vi "CN740_MODBUS_ASCII.vi"() -> ()   [LabVIEW 2023]
uses:
  <vilib>/Instr/_visa.llb/VISA Configure Serial Port (Instr).vi
panel:
  in  "Hysteresis 1":dbl=100.0 min=0.0 max=300.0 step=0.1 format="%.1f"
  out "Mode ON/OFF":bool
  out "Mode PID":bool
  in  "Switch  Mode":bool
  in  "SV 1":dbl=100.0 min=0.0 max=300.0 step=0.1 format="%.1f"
  out "PV 1":dbl format="%.1f"
  in  "DC Pulse (ON/OFF)":bool
  in  "VISA Controller 1":refnum<visa-resource-name>="COM6"
  in  "Hysteresis":dbl=100.0 min=0.0 max=300.0 step=0.1 format="%.1f"
  in  "Switch Mode":bool
  out "Mode ON/OFF":bool
  out "Mode PID":bool
  in  "DC Pulse (ON/OFF)":bool
  in  "VISA Controller 3":refnum<visa-resource-name>="COM6"
  in  "SV 3":dbl=100.0 min=0.0 max=300.0 step=0.1 format="%.1f"
  out "PV 3":dbl format="%.1f"
  out "Mode ON/OFF":bool
  out "Mode PID":bool
  in  "Switch  Mode":bool
  in  "SV 2":dbl=100.0 min=0.0 max=300.0 step=0.1 format="%.1f"
  out "PV 2":dbl format="%.1f"
  in  "DC Pulse (ON/OFF)":bool
  in  "Hysteresis":dbl=100.0 min=0.0 max=300.0 step=0.1 format="%.1f"
  in  "VISA Controller 2":refnum<visa-resource-name>="COM6"
  in  "stop":bool
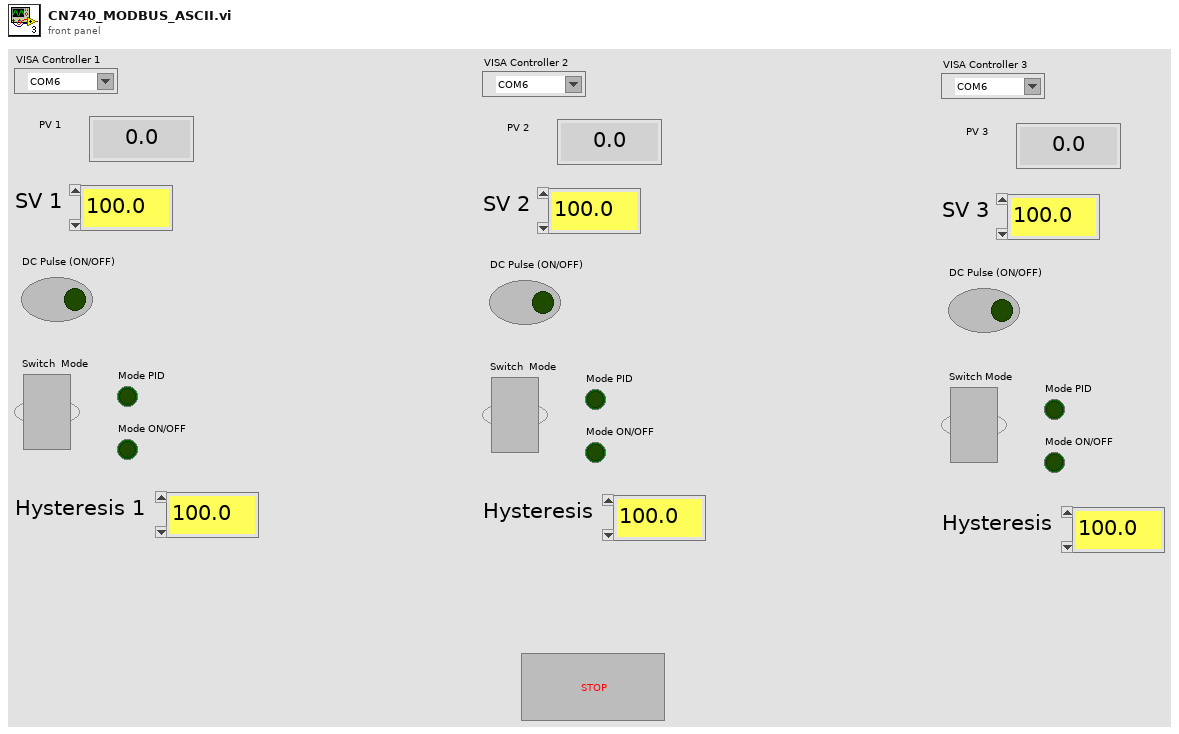
[diagram p1: front panel]
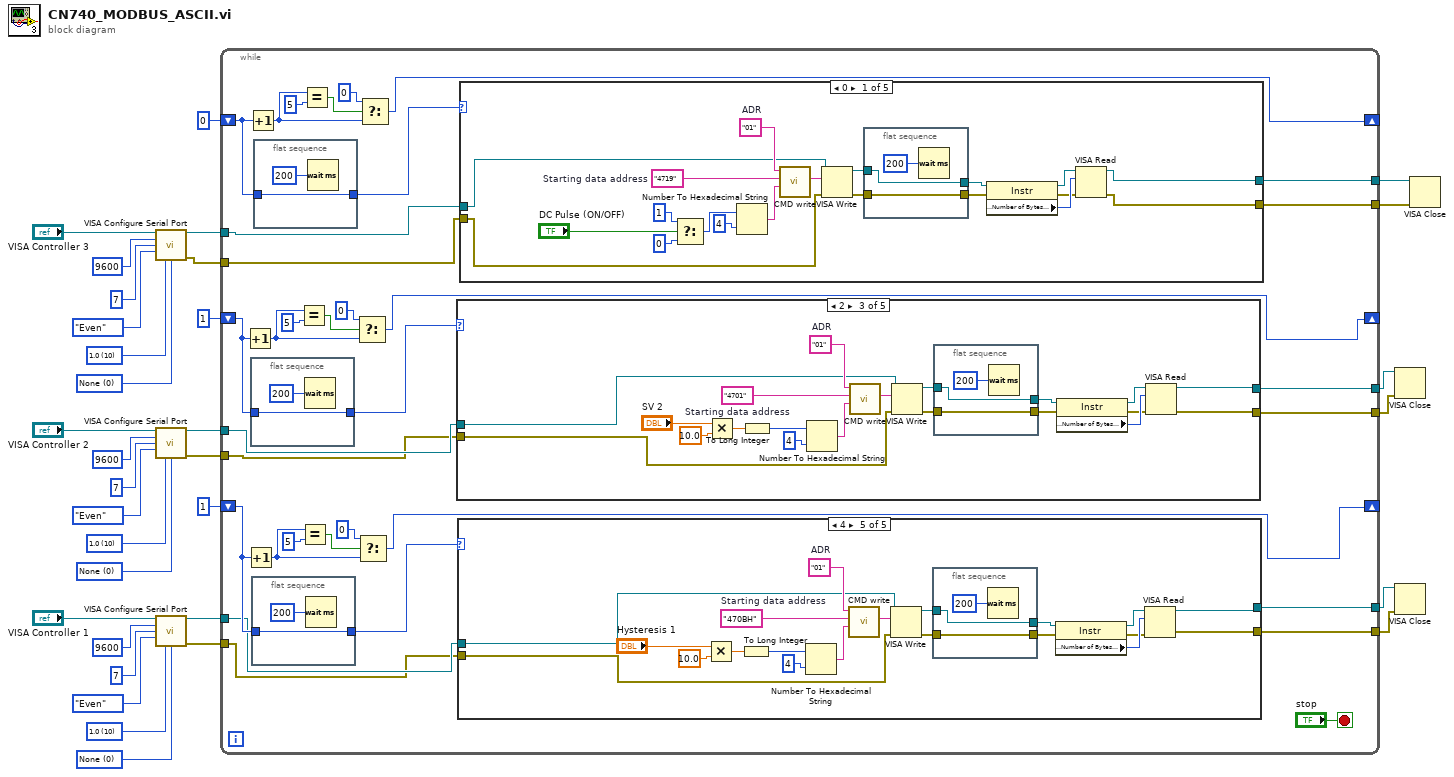
[diagram p0: block diagram]
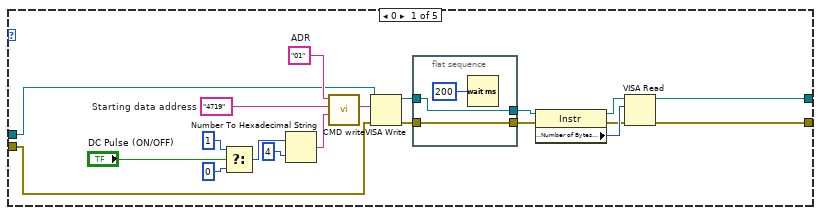
[diagram p2: hidden frame]
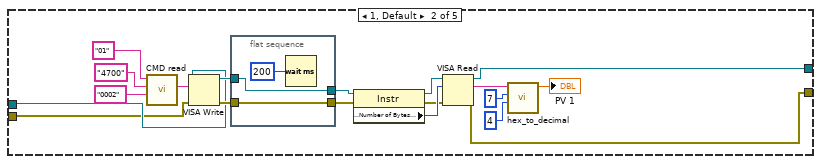
[diagram p3: hidden frame]
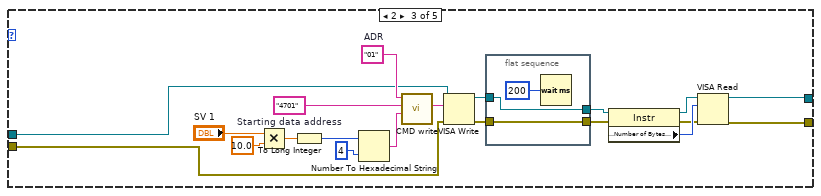
[diagram p4: hidden frame]
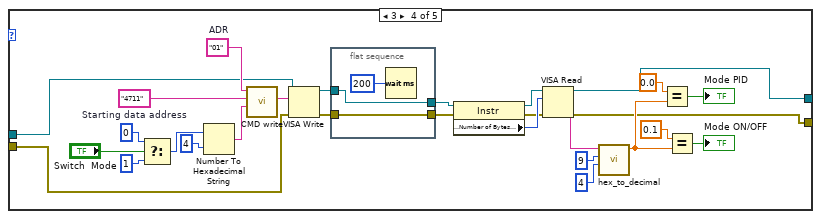
[diagram p5: hidden frame]
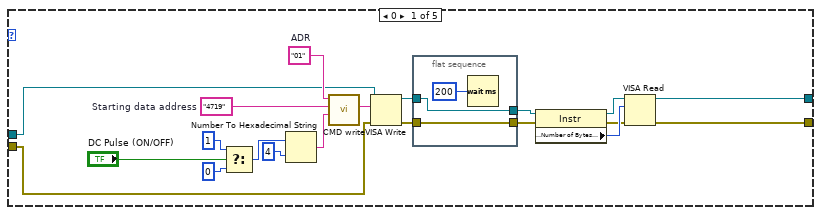
[diagram p6: hidden frame]
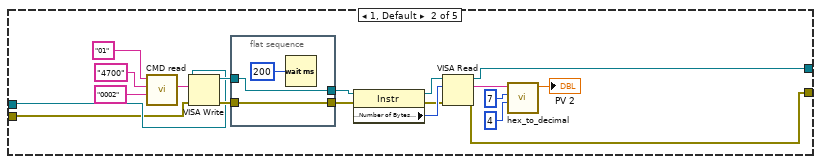
[diagram p7: hidden frame]
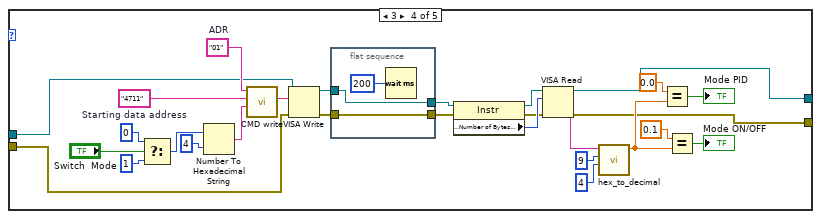
[diagram p8: hidden frame]
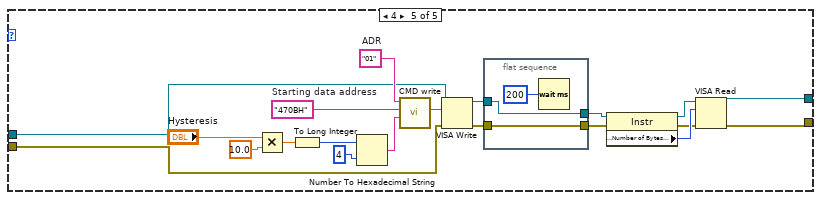
[diagram p9: hidden frame]
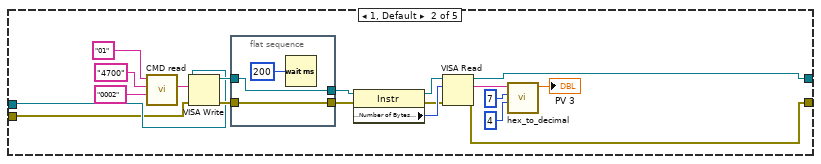
[diagram p10: hidden frame]
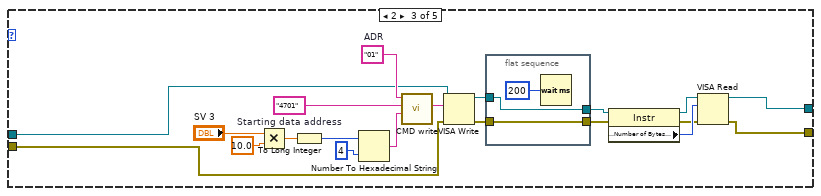
[diagram p11: hidden frame]
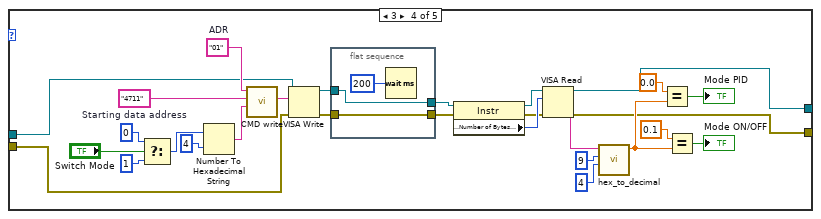
[diagram p12: hidden frame]
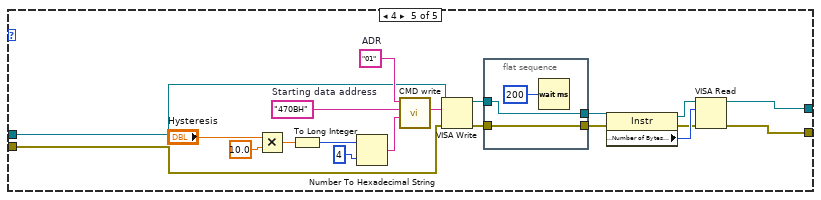
[diagram p13: hidden frame]
diagram:
  w10 = u16 0 items=["None"=0, "XON/XOFF"=1, "RTS/CTS"=2, "DTR/DSR"=4] ("flow control (0:none)")
  w11 = u16 10 items=["1.0"=10, "1.5"=15, "2.0"=20] ("stop bits (10: 1 bit)")
  w19 = u16 0 items=["None"=0, "XON/XOFF"=1, "RTS/CTS"=2, "DTR/DSR"=4] ("flow control (0:none)")
  w20 = u16 10 items=["1.0"=10, "1.5"=15, "2.0"=20] ("stop bits (10: 1 bit)")
  w28 = u16 0 items=["None"=0, "XON/XOFF"=1, "RTS/CTS"=2, "DTR/DSR"=4] ("flow control (0:none)")
  w29 = u16 10 items=["1.0"=10, "1.5"=15, "2.0"=20] ("stop bits (10: 1 bit)")
  n1 = call-poly "VISA Configure Serial Port"("VISA resource name"="VISA Controller 3", "baud rate (9600)"=u32 9600, "data bits (8)"=u16 7, "parity (0:none)"=enum16{"None", "Odd", "Even", "Mark", "Space"}."Even", "stop bits (10: 1 bit)"=w11, "flow control (0:none)"=w10) -> ("VISA resource name out"=w9:refnum<visa-resource-name>, "error out"=w8:errorcluster)  [unwired: 2 in, 6 out]
  n2 = call-poly "VISA Configure Serial Port"("VISA resource name"="VISA Controller 2", "baud rate (9600)"=u32 9600, "data bits (8)"=u16 7, "parity (0:none)"=enum16{"None", "Odd", "Even", "Mark", "Space"}."Even", "stop bits (10: 1 bit)"=w20, "flow control (0:none)"=w19) -> ("VISA resource name out"=w17:refnum<visa-resource-name>, "error out"=w18:errorcluster)  [unwired: 2 in, 6 out]
  n3 = call-poly "VISA Configure Serial Port"("VISA resource name"="VISA Controller 1", "baud rate (9600)"=u32 9600, "data bits (8)"=u16 7, "parity (0:none)"=enum16{"None", "Odd", "Even", "Mark", "Space"}."Even", "stop bits (10: 1 bit)"=w29, "flow control (0:none)"=w28) -> ("VISA resource name out"=w27:refnum<visa-resource-name>, "error out"=w26:errorcluster)  [unwired: 2 in, 6 out]
  n4 = while {
    tunnel: w26 -> [w40]
    tunnel: w27 -> [w41]
    shift-right: [w46] -> _
    shift-left: 1 -> [w44]
    tunnel: w18 -> [w42]
    tunnel: w17 -> [w43]
    shift-right: [w47] -> _
    shift-left: 1 -> [w45]
    tunnel: w9 -> [w61]
    tunnel: w8 -> [w60]
    shift-right: [w58] -> _
    shift-left: 0 -> [w59]
    tunnel: [w39] -> w6
    tunnel: [w38] -> w5
    tunnel: [w37] -> w4
    tunnel: [w36] -> w3
    tunnel: [w35] -> w2
    tunnel: [w34] -> w1
    stop <- "stop" stop-if-true
    n5 = Increment(x=w45) -> (x+1=w55:i32)
    n6 = Increment(x=w44) -> (x+1=w50:i32)
    n7 = Increment(x=w59) -> (x+1=w64:i32)
    n8 = flat-sequence {
      tunnel: w45 -> [w192]
      tunnel: [w192] -> w53
      frame #0 {
        n9 = Wait (ms)(milliseconds to wait=u32 200 ("attente (ms)")) -> ()  [unwired: 1 out]
      }
    }
    n10 = flat-sequence {
      tunnel: w44 -> [w68]
      tunnel: [w68] -> w48
      frame #0 {
        n11 = Wait (ms)(milliseconds to wait=u32 200 ("attente (ms)")) -> ()  [unwired: 1 out]
      }
    }
    n12 = flat-sequence {
      tunnel: w59 -> [w316]
      tunnel: [w316] -> w62
      frame #0 {
        n13 = Wait (ms)(milliseconds to wait=u32 200 ("attente (ms)")) -> ()  [unwired: 1 out]
      }
    }
    n14 = Equal?(x=w55, y=5) -> (x = y?=w56:bool)
    n15 = Equal?(x=w50, y=5) -> (x = y?=w51:bool)
    n16 = Equal?(x=w64, y=5) -> (x = y?=w65:bool)
    n17 = Select(t=0, s=w56, f=w55) -> (s? t:f=w47:i32)
    n18 = Select(t=0, s=w51, f=w50) -> (s? t:f=w46:i32)
    n19 = Select(t=0, s=w65, f=w64) -> (s? t:f=w58:i32)
    n20 = case shown="2" w53 {
      tunnel: w43 -> [w197 w220 w242 w274 w296]
      tunnel: w42 -> [w196 w219 w241 w273 w295]
      tunnel: [w195 w218 w240 w263 w293] -> w37
      tunnel: [w194 w217 w239 w262 w294] -> w36
      frame 0 {
        w206 = "01"  # ADR
        w205 = "4719"  # Starting data address
        n21 = Select(t=1, s="DC Pulse (ON/OFF)", f=0) -> (s? t:f=w200:i32)
        n22 = Number To Hexadecimal String(1:i16 4 ("largeur (-)"), 2:w200) -> (0:w198:string)
        n23 = call "CMD write.vi"("Data Content"=w198, "Starting data address"=w205, "ADR"=w206) -> ("Chaîne en sortie"=w204:string)  [unwired: 6 in]
        n24 = VISA Write(VISA resource name=w197, write buffer=w204, error in (no error)=w196) -> (VISA resource name out=w210:refnum<visa-resource-name>, error out=w207:errorcluster)  [unwired: 1 out]
        n25 = flat-sequence {
          tunnel: w210 -> [w215]
          tunnel: [w215] -> w209
          tunnel: [w214] -> w208
          tunnel: w207 -> [w214]
          frame #0 {
            n26 = Wait (ms)(milliseconds to wait=u32 200 ("attente (ms)")) -> ()  [unwired: 1 out]
          }
        }
        n27 = property class="Instr"(reference=w209, error in=w208) -> (reference out=w213:refnum<visa-resource-name>, error out=w211:errorcluster, "Serial Settings:Number of Bytes at Serial Port"=w212:u32)
        n28 = VISA Read(VISA resource name=w213, byte count=w212, error in (no error)=w211) -> (VISA resource name out=w195:refnum<visa-resource-name>, error out=w194:errorcluster)  [unwired: 2 out]
      }
      frame 1, Default {
        n29 = call "CMD read.vi"("Data Content"="0002", "Starting data address"="4700", "ADR"="01") -> ("Chaîne en sortie"=w222:string)  [unwired: 6 in]
        n30 = VISA Write(VISA resource name=w220, write buffer=w222, error in (no error)=w219) -> (VISA resource name out=w232:refnum<visa-resource-name>, error out=w229:errorcluster)  [unwired: 1 out]
        n31 = flat-sequence {
          tunnel: w232 -> [w237]
          tunnel: [w237] -> w231
          tunnel: [w236] -> w230
          tunnel: w229 -> [w236]
          frame #0 {
            n32 = Wait (ms)(milliseconds to wait=u32 200 ("attente (ms)")) -> ()  [unwired: 1 out]
          }
        }
        n33 = property class="Instr"(reference=w231, error in=w230) -> (reference out=w235:refnum<visa-resource-name>, error out=w233:errorcluster, "Serial Settings:Number of Bytes at Serial Port"=w234:u32)
        n34 = VISA Read(VISA resource name=w235, byte count=w234, error in (no error)=w233) -> (VISA resource name out=w218:refnum<visa-resource-name>, read buffer=w221:string, error out=w217:errorcluster)  [unwired: 1 out]
        n35 = call "hex_to_decimal.vi"("length (rest)"=4, "offset (0)"=7, "read buffer"=w221) -> ("Numeric"=→"PV 2":dbl)  [unwired: 8 in]
      }
      frame 2 {
        w246 = "01"  # ADR
        w244 = "4701"  # Starting data address
        n36 = Multiply(x="SV 2", y=10.0) -> (x*y=w254:dbl)
        n37 = To Long Integer(number=w254) -> (32bit integer=w258:i32)
        n38 = Number To Hexadecimal String(1:i16 4 ("largeur (-)"), 2:w258) -> (0:w245:string)
        n39 = call "CMD write.vi"("Data Content"=w245, "Starting data address"=w244, "ADR"=w246) -> ("Chaîne en sortie"=w243:string)  [unwired: 6 in]
        n40 = VISA Write(VISA resource name=w242, write buffer=w243, error in (no error)=w241) -> (VISA resource name out=w250:refnum<visa-resource-name>, error out=w247:errorcluster)  [unwired: 1 out]
        n41 = flat-sequence {
          tunnel: w250 -> [w260]
          tunnel: [w260] -> w249
          tunnel: [w259] -> w248
          tunnel: w247 -> [w259]
          frame #0 {
            n42 = Wait (ms)(milliseconds to wait=u32 200 ("attente (ms)")) -> ()  [unwired: 1 out]
          }
        }
        n43 = property class="Instr"(reference=w249, error in=w248) -> (reference out=w253:refnum<visa-resource-name>, error out=w251:errorcluster, "Serial Settings:Number of Bytes at Serial Port"=w252:u32)
        n44 = VISA Read(VISA resource name=w253, byte count=w252, error in (no error)=w251) -> (VISA resource name out=w240:refnum<visa-resource-name>, error out=w239:errorcluster)  [unwired: 2 out]
      }
      frame 3 {
        w282 = "01"  # ADR
        w281 = "4711"  # Starting data address
        n45 = Select(t=0, s="Switch  Mode", f=1) -> (s? t:f=w277:i32)
        n46 = Number To Hexadecimal String(1:i16 4 ("largeur (-)"), 2:w277) -> (0:w275:string)
        n47 = call "CMD write.vi"("Data Content"=w275, "Starting data address"=w281, "ADR"=w282) -> ("Chaîne en sortie"=w280:string)  [unwired: 6 in]
        n48 = VISA Write(VISA resource name=w274, write buffer=w280, error in (no error)=w273) -> (VISA resource name out=w286:refnum<visa-resource-name>, error out=w283:errorcluster)  [unwired: 1 out]
        n49 = flat-sequence {
          tunnel: w286 -> [w291]
          tunnel: [w291] -> w285
          tunnel: [w290] -> w284
          tunnel: w283 -> [w290]
          frame #0 {
            n50 = Wait (ms)(milliseconds to wait=u32 200 ("attente (ms)")) -> ()  [unwired: 1 out]
          }
        }
        n51 = property class="Instr"(reference=w285, error in=w284) -> (reference out=w289:refnum<visa-resource-name>, error out=w287:errorcluster, "Serial Settings:Number of Bytes at Serial Port"=w288:u32)
        n52 = VISA Read(VISA resource name=w289, byte count=w288, error in (no error)=w287) -> (VISA resource name out=w263:refnum<visa-resource-name>, read buffer=w270:string, error out=w262:errorcluster)  [unwired: 1 out]
        n53 = call "hex_to_decimal.vi"("length (rest)"=4, "offset (0)"=9, "read buffer"=w270) -> ("Numeric"=w268:dbl)  [unwired: 8 in]
        n54 = Equal?(x=0.0, y=w268) -> (x = y?=→"Mode PID":bool)
        n55 = Equal?(x=0.1, y=w268) -> (x = y?=→"Mode ON/OFF":bool)
      }
      frame 4 {
        w300 = "01"  # ADR
        w298 = "470BH"  # Starting data address
        n56 = Multiply(x="Hysteresis", y=10.0) -> (x*y=w308:dbl)
        n57 = To Long Integer(number=w308) -> (32bit integer=w312:i32)
        n58 = Number To Hexadecimal String(1:i16 4 ("largeur (-)"), 2:w312) -> (0:w299:string)
        n59 = call "CMD write.vi"("Data Content"=w299, "Starting data address"=w298, "ADR"=w300) -> ("Chaîne en sortie"=w297:string)  [unwired: 6 in]
        n60 = VISA Write(VISA resource name=w296, write buffer=w297, error in (no error)=w295) -> (VISA resource name out=w304:refnum<visa-resource-name>, error out=w301:errorcluster)  [unwired: 1 out]
        n61 = flat-sequence {
          tunnel: w304 -> [w314]
          tunnel: [w314] -> w303
          tunnel: [w313] -> w302
          tunnel: w301 -> [w313]
          frame #0 {
            n62 = Wait (ms)(milliseconds to wait=u32 200 ("attente (ms)")) -> ()  [unwired: 1 out]
          }
        }
        n63 = property class="Instr"(reference=w303, error in=w302) -> (reference out=w307:refnum<visa-resource-name>, error out=w305:errorcluster, "Serial Settings:Number of Bytes at Serial Port"=w306:u32)
        n64 = VISA Read(VISA resource name=w307, byte count=w306, error in (no error)=w305) -> (VISA resource name out=w293:refnum<visa-resource-name>, error out=w294:errorcluster)  [unwired: 2 out]
      }
    }
    n65 = case shown="4" w48 {
      tunnel: w41 -> [w73 w96 w118 w150 w172]
      tunnel: w40 -> [w72 w95 w117 w149 w171]
      tunnel: [w71 w94 w116 w139 w170] -> w35
      tunnel: [w70 w93 w115 w138 w169] -> w34
      frame 0 {
        w82 = "01"  # ADR
        w81 = "4719"  # Starting data address
        n66 = Select(t=1, s="DC Pulse (ON/OFF)", f=0) -> (s? t:f=w76:i32)
        n67 = Number To Hexadecimal String(1:i16 4 ("largeur (-)"), 2:w76) -> (0:w74:string)
        n68 = call "CMD write.vi"("Data Content"=w74, "Starting data address"=w81, "ADR"=w82) -> ("Chaîne en sortie"=w80:string)  [unwired: 6 in]
        n69 = VISA Write(VISA resource name=w73, write buffer=w80, error in (no error)=w72) -> (VISA resource name out=w86:refnum<visa-resource-name>, error out=w83:errorcluster)  [unwired: 1 out]
        n70 = flat-sequence {
          tunnel: w86 -> [w91]
          tunnel: [w91] -> w85
          tunnel: [w90] -> w84
          tunnel: w83 -> [w90]
          frame #0 {
            n71 = Wait (ms)(milliseconds to wait=u32 200 ("attente (ms)")) -> ()  [unwired: 1 out]
          }
        }
        n72 = property class="Instr"(reference=w85, error in=w84) -> (reference out=w89:refnum<visa-resource-name>, error out=w87:errorcluster, "Serial Settings:Number of Bytes at Serial Port"=w88:u32)
        n73 = VISA Read(VISA resource name=w89, byte count=w88, error in (no error)=w87) -> (VISA resource name out=w71:refnum<visa-resource-name>, error out=w70:errorcluster)  [unwired: 2 out]
      }
      frame 1, Default {
        n74 = call "CMD read.vi"("Data Content"="0002", "Starting data address"="4700", "ADR"="01") -> ("Chaîne en sortie"=w98:string)  [unwired: 6 in]
        n75 = VISA Write(VISA resource name=w96, write buffer=w98, error in (no error)=w95) -> (VISA resource name out=w108:refnum<visa-resource-name>, error out=w105:errorcluster)  [unwired: 1 out]
        n76 = flat-sequence {
          tunnel: w108 -> [w113]
          tunnel: [w113] -> w107
          tunnel: [w112] -> w106
          tunnel: w105 -> [w112]
          frame #0 {
            n77 = Wait (ms)(milliseconds to wait=u32 200 ("attente (ms)")) -> ()  [unwired: 1 out]
          }
        }
        n78 = property class="Instr"(reference=w107, error in=w106) -> (reference out=w111:refnum<visa-resource-name>, error out=w109:errorcluster, "Serial Settings:Number of Bytes at Serial Port"=w110:u32)
        n79 = VISA Read(VISA resource name=w111, byte count=w110, error in (no error)=w109) -> (VISA resource name out=w94:refnum<visa-resource-name>, read buffer=w97:string, error out=w93:errorcluster)  [unwired: 1 out]
        n80 = call "hex_to_decimal.vi"("length (rest)"=4, "offset (0)"=7, "read buffer"=w97) -> ("Numeric"=→"PV 1":dbl)  [unwired: 8 in]
      }
      frame 2 {
        w122 = "01"  # ADR
        w120 = "4701"  # Starting data address
        n81 = Multiply(x="SV 1", y=10.0) -> (x*y=w130:dbl)
        n82 = To Long Integer(number=w130) -> (32bit integer=w134:i32)
        n83 = Number To Hexadecimal String(1:i16 4 ("largeur (-)"), 2:w134) -> (0:w121:string)
        n84 = call "CMD write.vi"("Data Content"=w121, "Starting data address"=w120, "ADR"=w122) -> ("Chaîne en sortie"=w119:string)  [unwired: 6 in]
        n85 = VISA Write(VISA resource name=w118, write buffer=w119, error in (no error)=w117) -> (VISA resource name out=w126:refnum<visa-resource-name>, error out=w123:errorcluster)  [unwired: 1 out]
        n86 = flat-sequence {
          tunnel: w126 -> [w136]
          tunnel: [w136] -> w125
          tunnel: [w135] -> w124
          tunnel: w123 -> [w135]
          frame #0 {
            n87 = Wait (ms)(milliseconds to wait=u32 200 ("attente (ms)")) -> ()  [unwired: 1 out]
          }
        }
        n88 = property class="Instr"(reference=w125, error in=w124) -> (reference out=w129:refnum<visa-resource-name>, error out=w127:errorcluster, "Serial Settings:Number of Bytes at Serial Port"=w128:u32)
        n89 = VISA Read(VISA resource name=w129, byte count=w128, error in (no error)=w127) -> (VISA resource name out=w116:refnum<visa-resource-name>, error out=w115:errorcluster)  [unwired: 2 out]
      }
      frame 3 {
        w158 = "01"  # ADR
        w157 = "4711"  # Starting data address
        n90 = Select(t=0, s="Switch  Mode", f=1) -> (s? t:f=w153:i32)
        n91 = Number To Hexadecimal String(1:i16 4 ("largeur (-)"), 2:w153) -> (0:w151:string)
        n92 = call "CMD write.vi"("Data Content"=w151, "Starting data address"=w157, "ADR"=w158) -> ("Chaîne en sortie"=w156:string)  [unwired: 6 in]
        n93 = VISA Write(VISA resource name=w150, write buffer=w156, error in (no error)=w149) -> (VISA resource name out=w162:refnum<visa-resource-name>, error out=w159:errorcluster)  [unwired: 1 out]
        n94 = flat-sequence {
          tunnel: w162 -> [w167]
          tunnel: [w167] -> w161
          tunnel: [w166] -> w160
          tunnel: w159 -> [w166]
          frame #0 {
            n95 = Wait (ms)(milliseconds to wait=u32 200 ("attente (ms)")) -> ()  [unwired: 1 out]
          }
        }
        n96 = property class="Instr"(reference=w161, error in=w160) -> (reference out=w165:refnum<visa-resource-name>, error out=w163:errorcluster, "Serial Settings:Number of Bytes at Serial Port"=w164:u32)
        n97 = VISA Read(VISA resource name=w165, byte count=w164, error in (no error)=w163) -> (VISA resource name out=w139:refnum<visa-resource-name>, read buffer=w146:string, error out=w138:errorcluster)  [unwired: 1 out]
        n98 = call "hex_to_decimal.vi"("length (rest)"=4, "offset (0)"=9, "read buffer"=w146) -> ("Numeric"=w144:dbl)  [unwired: 8 in]
        n99 = Equal?(x=0.0, y=w144) -> (x = y?=→"Mode PID":bool)
        n100 = Equal?(x=0.1, y=w144) -> (x = y?=→"Mode ON/OFF":bool)
      }
      frame 4 {
        w176 = "01"  # ADR
        w174 = "470BH"  # Starting data address
        n101 = Multiply(x="Hysteresis 1", y=10.0) -> (x*y=w184:dbl)
        n102 = To Long Integer(number=w184) -> (32bit integer=w188:i32)
        n103 = Number To Hexadecimal String(1:i16 4 ("largeur (-)"), 2:w188) -> (0:w175:string)
        n104 = call "CMD write.vi"("Data Content"=w175, "Starting data address"=w174, "ADR"=w176) -> ("Chaîne en sortie"=w173:string)  [unwired: 6 in]
        n105 = VISA Write(VISA resource name=w172, write buffer=w173, error in (no error)=w171) -> (VISA resource name out=w180:refnum<visa-resource-name>, error out=w177:errorcluster)  [unwired: 1 out]
        n106 = flat-sequence {
          tunnel: w180 -> [w190]
          tunnel: [w190] -> w179
          tunnel: [w189] -> w178
          tunnel: w177 -> [w189]
          frame #0 {
            n107 = Wait (ms)(milliseconds to wait=u32 200 ("attente (ms)")) -> ()  [unwired: 1 out]
          }
        }
        n108 = property class="Instr"(reference=w179, error in=w178) -> (reference out=w183:refnum<visa-resource-name>, error out=w181:errorcluster, "Serial Settings:Number of Bytes at Serial Port"=w182:u32)
        n109 = VISA Read(VISA resource name=w183, byte count=w182, error in (no error)=w181) -> (VISA resource name out=w170:refnum<visa-resource-name>, error out=w169:errorcluster)  [unwired: 2 out]
      }
    }
    n110 = case shown="0" w62 {
      tunnel: w61 -> [w321 w344 w366 w398 w420]
      tunnel: w60 -> [w320 w343 w365 w397 w419]
      tunnel: [w319 w342 w364 w387 w418] -> w39
      tunnel: [w318 w341 w363 w386 w417] -> w38
      frame 0 {
        w330 = "01"  # ADR
        w329 = "4719"  # Starting data address
        n111 = Select(t=1, s="DC Pulse (ON/OFF)", f=0) -> (s? t:f=w324:i32)
        n112 = Number To Hexadecimal String(1:i16 4 ("largeur (-)"), 2:w324) -> (0:w322:string)
        n113 = call "CMD write.vi"("Data Content"=w322, "Starting data address"=w329, "ADR"=w330) -> ("Chaîne en sortie"=w328:string)  [unwired: 6 in]
        n114 = VISA Write(VISA resource name=w321, write buffer=w328, error in (no error)=w320) -> (VISA resource name out=w334:refnum<visa-resource-name>, error out=w331:errorcluster)  [unwired: 1 out]
        n115 = flat-sequence {
          tunnel: w334 -> [w339]
          tunnel: [w339] -> w333
          tunnel: [w338] -> w332
          tunnel: w331 -> [w338]
          frame #0 {
            n116 = Wait (ms)(milliseconds to wait=u32 200 ("attente (ms)")) -> ()  [unwired: 1 out]
          }
        }
        n117 = property class="Instr"(reference=w333, error in=w332) -> (reference out=w337:refnum<visa-resource-name>, error out=w335:errorcluster, "Serial Settings:Number of Bytes at Serial Port"=w336:u32)
        n118 = VISA Read(VISA resource name=w337, byte count=w336, error in (no error)=w335) -> (VISA resource name out=w319:refnum<visa-resource-name>, error out=w318:errorcluster)  [unwired: 2 out]
      }
      frame 1, Default {
        n119 = call "CMD read.vi"("Data Content"="0002", "Starting data address"="4700", "ADR"="01") -> ("Chaîne en sortie"=w346:string)  [unwired: 6 in]
        n120 = VISA Write(VISA resource name=w344, write buffer=w346, error in (no error)=w343) -> (VISA resource name out=w356:refnum<visa-resource-name>, error out=w353:errorcluster)  [unwired: 1 out]
        n121 = flat-sequence {
          tunnel: w356 -> [w361]
          tunnel: [w361] -> w355
          tunnel: [w360] -> w354
          tunnel: w353 -> [w360]
          frame #0 {
            n122 = Wait (ms)(milliseconds to wait=u32 200 ("attente (ms)")) -> ()  [unwired: 1 out]
          }
        }
        n123 = property class="Instr"(reference=w355, error in=w354) -> (reference out=w359:refnum<visa-resource-name>, error out=w357:errorcluster, "Serial Settings:Number of Bytes at Serial Port"=w358:u32)
        n124 = VISA Read(VISA resource name=w359, byte count=w358, error in (no error)=w357) -> (VISA resource name out=w342:refnum<visa-resource-name>, read buffer=w345:string, error out=w341:errorcluster)  [unwired: 1 out]
        n125 = call "hex_to_decimal.vi"("length (rest)"=4, "offset (0)"=7, "read buffer"=w345) -> ("Numeric"=→"PV 3":dbl)  [unwired: 8 in]
      }
      frame 2 {
        w370 = "01"  # ADR
        w368 = "4701"  # Starting data address
        n126 = Multiply(x="SV 3", y=10.0) -> (x*y=w378:dbl)
        n127 = To Long Integer(number=w378) -> (32bit integer=w382:i32)
        n128 = Number To Hexadecimal String(1:i16 4 ("largeur (-)"), 2:w382) -> (0:w369:string)
        n129 = call "CMD write.vi"("Data Content"=w369, "Starting data address"=w368, "ADR"=w370) -> ("Chaîne en sortie"=w367:string)  [unwired: 6 in]
        n130 = VISA Write(VISA resource name=w366, write buffer=w367, error in (no error)=w365) -> (VISA resource name out=w374:refnum<visa-resource-name>, error out=w371:errorcluster)  [unwired: 1 out]
        n131 = flat-sequence {
          tunnel: w374 -> [w384]
          tunnel: [w384] -> w373
          tunnel: [w383] -> w372
          tunnel: w371 -> [w383]
          frame #0 {
            n132 = Wait (ms)(milliseconds to wait=u32 200 ("attente (ms)")) -> ()  [unwired: 1 out]
          }
        }
        n133 = property class="Instr"(reference=w373, error in=w372) -> (reference out=w377:refnum<visa-resource-name>, error out=w375:errorcluster, "Serial Settings:Number of Bytes at Serial Port"=w376:u32)
        n134 = VISA Read(VISA resource name=w377, byte count=w376, error in (no error)=w375) -> (VISA resource name out=w364:refnum<visa-resource-name>, error out=w363:errorcluster)  [unwired: 2 out]
      }
      frame 3 {
        w406 = "01"  # ADR
        w405 = "4711"  # Starting data address
        n135 = Select(t=0, s="Switch Mode", f=1) -> (s? t:f=w401:i32)
        n136 = Number To Hexadecimal String(1:i16 4 ("largeur (-)"), 2:w401) -> (0:w399:string)
        n137 = call "CMD write.vi"("Data Content"=w399, "Starting data address"=w405, "ADR"=w406) -> ("Chaîne en sortie"=w404:string)  [unwired: 6 in]
        n138 = VISA Write(VISA resource name=w398, write buffer=w404, error in (no error)=w397) -> (VISA resource name out=w410:refnum<visa-resource-name>, error out=w407:errorcluster)  [unwired: 1 out]
        n139 = flat-sequence {
          tunnel: w410 -> [w415]
          tunnel: [w415] -> w409
          tunnel: [w414] -> w408
          tunnel: w407 -> [w414]
          frame #0 {
            n140 = Wait (ms)(milliseconds to wait=u32 200 ("attente (ms)")) -> ()  [unwired: 1 out]
          }
        }
        n141 = property class="Instr"(reference=w409, error in=w408) -> (reference out=w413:refnum<visa-resource-name>, error out=w411:errorcluster, "Serial Settings:Number of Bytes at Serial Port"=w412:u32)
        n142 = VISA Read(VISA resource name=w413, byte count=w412, error in (no error)=w411) -> (VISA resource name out=w387:refnum<visa-resource-name>, read buffer=w394:string, error out=w386:errorcluster)  [unwired: 1 out]
        n143 = call "hex_to_decimal.vi"("length (rest)"=4, "offset (0)"=9, "read buffer"=w394) -> ("Numeric"=w392:dbl)  [unwired: 8 in]
        n144 = Equal?(x=0.0, y=w392) -> (x = y?=→"Mode PID":bool)
        n145 = Equal?(x=0.1, y=w392) -> (x = y?=→"Mode ON/OFF":bool)
      }
      frame 4 {
        w424 = "01"  # ADR
        w422 = "470BH"  # Starting data address
        n146 = Multiply(x="Hysteresis", y=10.0) -> (x*y=w432:dbl)
        n147 = To Long Integer(number=w432) -> (32bit integer=w436:i32)
        n148 = Number To Hexadecimal String(1:i16 4 ("largeur (-)"), 2:w436) -> (0:w423:string)
        n149 = call "CMD write.vi"("Data Content"=w423, "Starting data address"=w422, "ADR"=w424) -> ("Chaîne en sortie"=w421:string)  [unwired: 6 in]
        n150 = VISA Write(VISA resource name=w420, write buffer=w421, error in (no error)=w419) -> (VISA resource name out=w428:refnum<visa-resource-name>, error out=w425:errorcluster)  [unwired: 1 out]
        n151 = flat-sequence {
          tunnel: w428 -> [w438]
          tunnel: [w438] -> w427
          tunnel: [w437] -> w426
          tunnel: w425 -> [w437]
          frame #0 {
            n152 = Wait (ms)(milliseconds to wait=u32 200 ("attente (ms)")) -> ()  [unwired: 1 out]
          }
        }
        n153 = property class="Instr"(reference=w427, error in=w426) -> (reference out=w431:refnum<visa-resource-name>, error out=w429:errorcluster, "Serial Settings:Number of Bytes at Serial Port"=w430:u32)
        n154 = VISA Read(VISA resource name=w431, byte count=w430, error in (no error)=w429) -> (VISA resource name out=w418:refnum<visa-resource-name>, error out=w417:errorcluster)  [unwired: 2 out]
      }
    }
  }
  n155 = VISA Close(VISA resource name=w4, error in (no error)=w3) -> ()  [unwired: 1 out]
  n156 = VISA Close(VISA resource name=w2, error in (no error)=w1) -> ()  [unwired: 1 out]
  n157 = VISA Close(VISA resource name=w6, error in (no error)=w5) -> ()  [unwired: 1 out]
